vi "Close Connection.vi"(0 "connection ID":refnum<k5>, 11 "error in (no error)":errorcluster) -> (15 "error out":errorcluster)   [LabVIEW 2014, in "hse-db.lvlib" / "MySQL (TCP).lvlib"]
uses:
  MySQL (TCP).lvlib
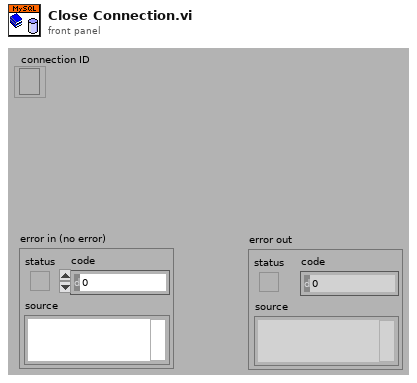
[diagram p1: front panel]
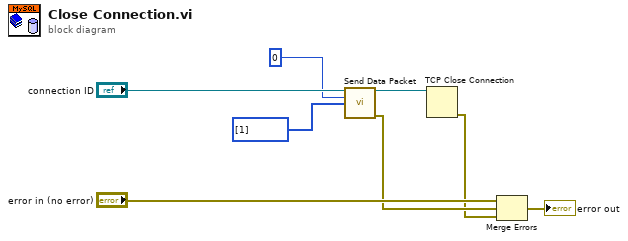
[diagram p0: block diagram]
diagram:
  n1 = call "Send Data Packet.vi"("connection ID"="connection ID", "Packet #"=u8 0, "TCP/IP Data"=u8[] [1]) -> ("connection ID out"=w5:refnum<k5>, "error out"=w3:errorcluster)  [unwired: 11 in]
  n2 = TCP Close Connection(connection ID=w5) -> (error out=w2:errorcluster)  [unwired: 2 in, 1 out]
  n3 = Merge Errors("error in (no error)", w3, w2) -> (→"error out":errorcluster)
